vi "Add Runtime Configurable Section.vi"(8 "error in":errorcluster, 11 "Node Ptr":u64 format="%.0x") -> (0 "error out":errorcluster)   [LabVIEW 2026, in "Runtime Configuration Support Example System Explorer.lvlib"]
uses:
  Runtime Configuration Support Example System Explorer.lvlib
  <vilib>/NI VeriStand/Custom Device API/Custom Device API.lvlib
panel:
  in  "Tag":string
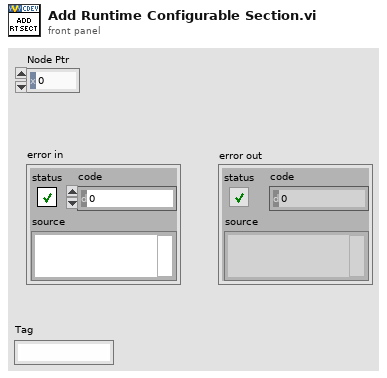
[diagram p1: front panel]
types:
  T1 = typedef "Custom Device API.lvlib/Custom Device Item Ref.ctl" = u64
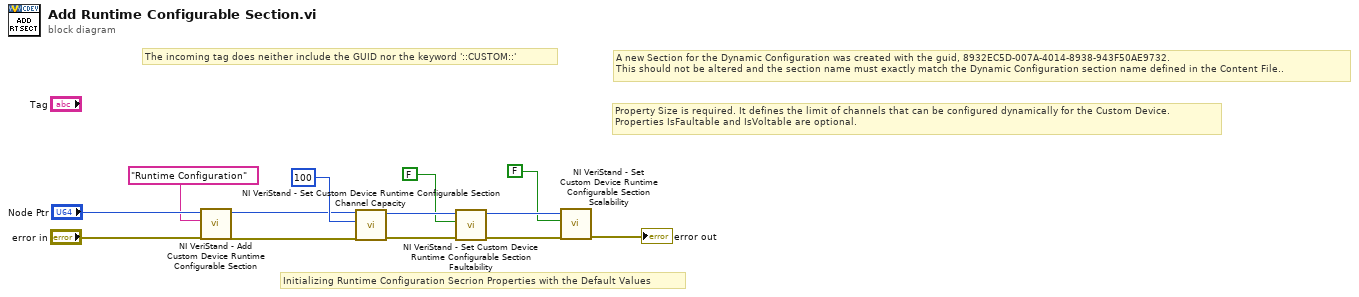
[diagram p0: block diagram]
diagram:
  # "Initializing Runtime Configuration Secrion Properties with the Default Values"
  # "Property Size is required. It defines the limit of channels that can be configured dynamically for the Custom Device.\nProperties IsFaultable and IsVoltable are optional."
  # "A new Section for the Dynamic Configuration was created with the guid, 8932EC5D-007A-4014-8938-943F50AE9732.\nThis should not be altered and the section name must exactly match the Dynamic Configuration section name defined in the Content File.."
  # "The incoming tag does neither include the GUID nor the keyword '::CUSTOM::'"
  n1 = call <vilib>:"NI VeriStand - Add Custom Device Runtime Configurable Section.vi"("error in"="error in", "Section Name"="Runtime Configuration", "Parent Ref in"="Node Ptr") -> ("error out"=w11:errorcluster, "Section Ptr"=w5:T1)  [unwired: 5 in, 2 out]
  n2 = call <vilib>:"NI VeriStand - Set Custom Device Runtime Configurable Section Channel Capacity.vi"("error in"=w11, "Reserved Channel Capacity"=100 ("Size"), "Parent Ref in"=w5) -> ("error out"=w10:errorcluster, "Parent Ref out"=w4:T1)  [unwired: 7 in]
  n3 = call <vilib>:"NI VeriStand - Set Custom Device Runtime Configurable Section Faultability.vi"("error in"=w10, "Faultable"=FALSE, "Parent Ref in"=w4) -> ("error out"=w9:errorcluster, "Parent Ref out"=w2:T1)  [unwired: 7 in]
  n4 = call <vilib>:"NI VeriStand - Set Custom Device Runtime Configurable Section Scalability.vi"("error in"=w9, "Scalable"=FALSE, "Parent Ref in"=w2) -> ("error out"=→"error out":errorcluster)  [unwired: 7 in, 1 out]
